vi "DetectTriggerGivenTrack.vi"(8 "error in (no error)":errorcluster, 9 "CameraFrame":i32, 10 "Track":T1, 11 "StimOnRailsThenOnTurns in":refnum<class "StimOnRailsThenOnTurns.lvclass">) -> (0 "error out":errorcluster, 2 "Triggered?":bool, 3 "StimOnRailsThenOnTurns out":refnum<class "StimOnRailsThenOnTurns.lvclass">)   [LabVIEW 2019, in "StimOnRailsThenOnTurns.lvclass"]
uses:
  DetectSuppressionDuration/StimOnRailsThenOnTurns.lvclass
  WormTrackCluster.ctl
  StimulusObject.lvclass
  TrackTerminationReasonEnum.ctl
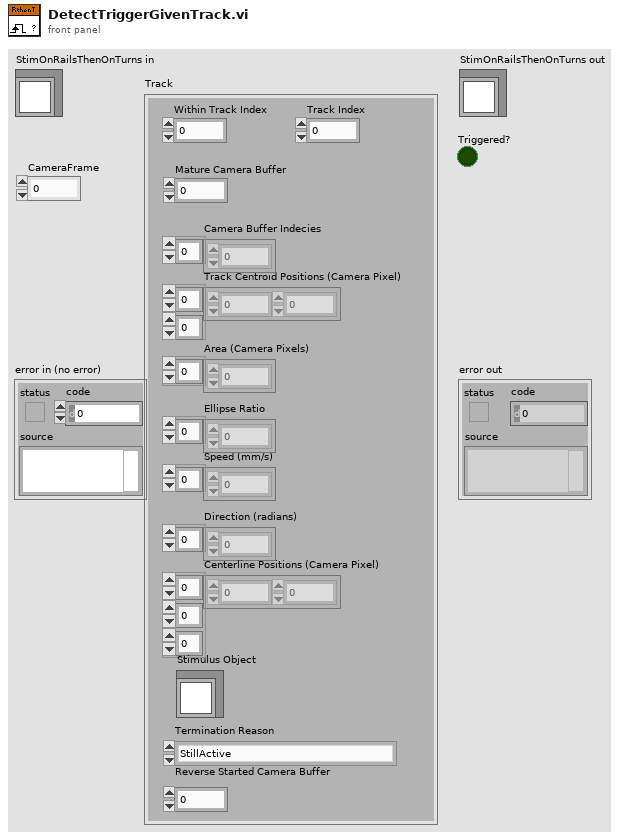
[diagram p1: front panel]
types:
  T1 = typedef "WormTrackCluster.ctl" = cluster{"Track Centroid Positions (Camera Pixel)":sgl[][], "Within Track Index":i32, "Camera Buffer Indecies":i32[], "Area (Camera Pixels)":i32[], "Speed (mm/s)":sgl[], "Direction (radians)":sgl[], "Centerline Positions (Camera Pixel)":sgl[][][], "Ellipse Ratio":sgl[], "Stimulus Object":refnum<class "StimulusObject.lvclass">, "Termination Reason":T2, "Track Index":i32, "Mature Camera Buffer":i32, "Reverse Started Camera Buffer":i32}
  T2 = typedef "TrackTerminationReasonEnum.ctl" = enum16{"StillActive", "MaxDisplacement", "NoBlobsLeft", "AreaIncrease", "AreaDecrease", "ExperimentEnded"}
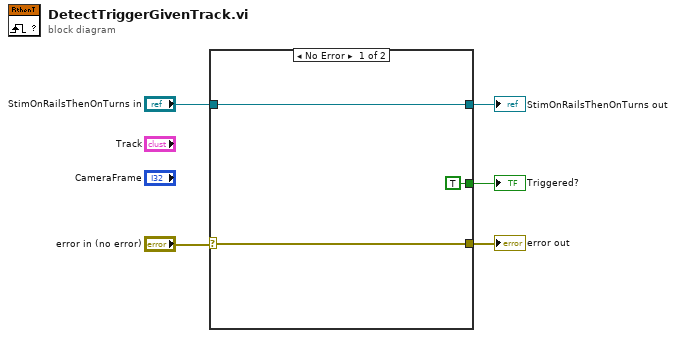
[diagram p0: block diagram]
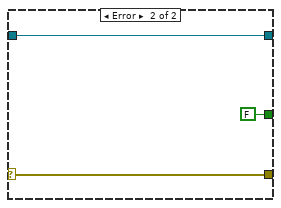
[diagram p2: hidden frame]
diagram:
  n1 = case shown="No Error" "error in (no error)" {
    selector: "error in (no error)" -> [w8 w10]
    tunnel: [w8 w10] -> w1
    tunnel: [w7 w11] -> w3
    tunnel: "StimOnRailsThenOnTurns in" -> [w7 w11]
    tunnel: [TRUE ("Triggered?") FALSE ("Triggered?")] -> w2
    frame No Error {
    }
    frame Error {
    }
  }
  "error out" <- w1
  "StimOnRailsThenOnTurns out" <- w3
  "Triggered?" <- w2
